vi "Get All Parameters.vi"(8 "error in (no error)":errorcluster, 11 "Assertion Step in":refnum<class "Assertion Step.lvclass">) -> (0 "error out":errorcluster, 2 "Parameters":T1={"Type"=enum."Mouse Move", "X"=0, "Y"=0, "Delay"=0, "Key"=65, "Repeat"=0, "RClick?"=FALSE, "App/Window Name"="", "Notes"="", "Assertion Type"=enum."Control Position", "Control Name"="", "Stop on Fail?"=FALSE, "Disabled"=enum."Enabled", "Visible"=enum."Visible", "Left"=0, "Top"=0, "Width"=0, "Height"=0, "Expected Image"={"image type"=0, "image depth"=0, "image"=[], "mask"=[], "colors"=[], "Rectangle"={"left"=0, "top"=0, "right"=0, "bottom"=0}}}, 3 "Assertion Step out":refnum<class "Assertion Step.lvclass">)   [LabVIEW 2020, in "MacroAssert.lvlib" / "Assertion Step.lvclass"]
uses:
  Assertion Step.lvclass
  Step/Step.lvclass
  Assertion Step.lvclass/Assertion Step.ctl
  CTLs/Step V3.ctl
  MacroAssert.lvlib
  CTLs/Step Type V3.ctl
  CTLs/Assertion Type.ctl
  <vilib>/picture/picture.llb/imagedata.ctl
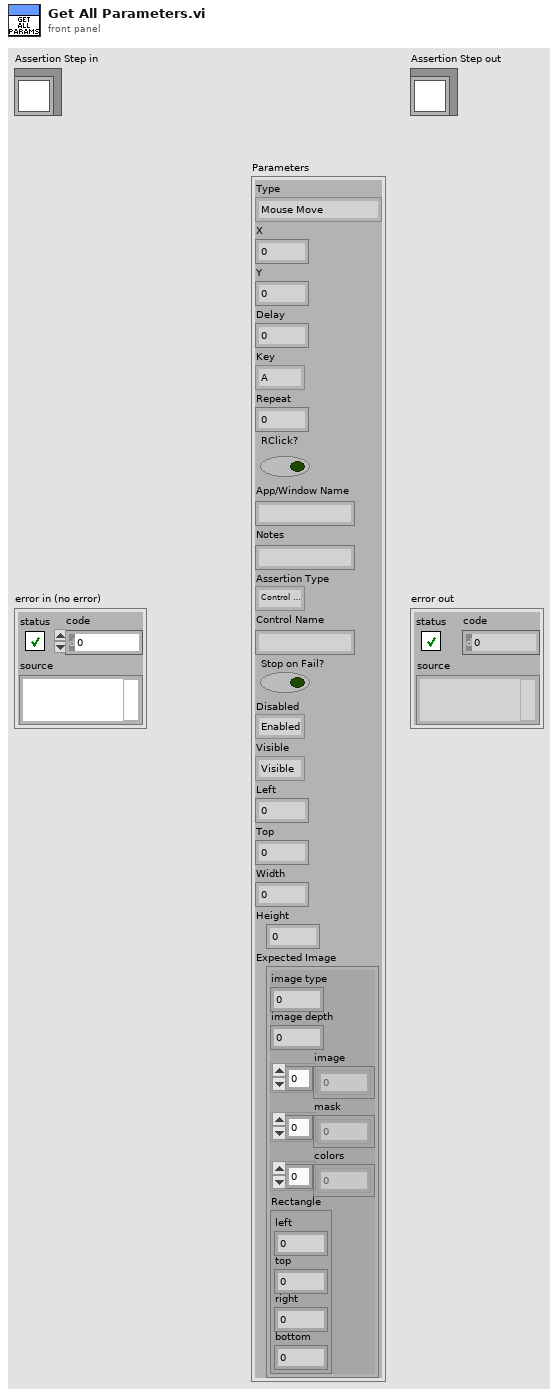
[diagram p1: front panel]
types:
  T1 = typedef "MacroAssert.lvlib/Step V3.ctl" = cluster{"Type":T2, "X":i32, "Y":i32, "Delay":i32, "Key":u8, "Repeat":i32, "RClick?":bool, "App/Window Name":string, "Notes":string, "Assertion Type":T3, "Control Name":string, "Stop on Fail?":bool, "Disabled":enum8{"Enabled", "Disabled", "Disabled and Grayed Out"}, "Visible":enum16{"Visible", "Not Visible"}, "Left":i16, "Top":i16, "Width":i16, "Height":i16, "Expected Image":T4}
  T2 = typedef "MacroAssert.lvlib/Step Type V3.ctl" = enum16{"Mouse Move", "Mouse Click", "Key Press", "Wait", "Mouse Down", "Mouse Up", "Key Down", "Key Up", "Maximize Window", "Restore Window", "Minimize Window", "Close Window", "Bring Window to Front", "Send Window to Back", "Assertion: Ctl Visible", "Assertion: Ctl Disabled", "Assertion: Ctl Image"}
  T3 = typedef "MacroAssert.lvlib/Assertion Type.ctl" = enum16{"Control Position", "Control Visible", "Control Disabled", "Control Image"}
  T4 = typedef "imagedata.ctl" = cluster{"image type":i32, "image depth":i32, "image":u8[], "mask":u8[], "colors":u32[], "Rectangle":cluster{"left":i16, "top":i16, "right":i16, "bottom":i16}}
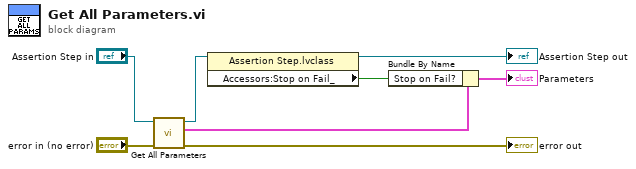
[diagram p0: block diagram]
diagram:
  n1 = call-parent "Get All Parameters.vi"("error in (no error)"="error in (no error)", "Step in"="Assertion Step in") -> ("error out"=→"error out":errorcluster, "Parameters"=w3:T1, "Step out"=w7:refnum<class "Assertion Step.lvclass">)  [unwired: 7 in]
  n2 = property class="Assertion Step.lvclass"(reference=w7) -> (reference out=→"Assertion Step out":refnum<class "Assertion Step.lvclass">, "Accessors:Stop on Fail_"=w1:bool)  [unwired: 1 in, 1 out]
  n3 = Bundle By Name(cluster=w3, "Stop on Fail?"=w1) -> (→"Parameters":T1)
